vi "general query.vi"(0 "VISA resource name":refnum<visa-resource-name>="GPIB0::21::INSTR", 11 "error in (no error)":errorcluster) -> (2 "Range W and dBm":T3, 3 "In Range?":T2, 4 "VISA resource name out":refnum<visa-resource-name>, 6 "Power":string, 8 "Power num":dbl, 10 "Units":string, 13 "Averaging":T4, 14 "Auto Ranging?":T1, 15 "error out":errorcluster)   [LabVIEW 2017]
uses:
  Averaging control.ctl
  Range control watts and dBm.ctl
  Range Status.ctl
  Auto Range control.ctl
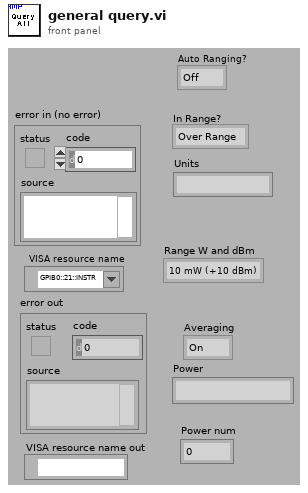
[diagram p1: front panel]
types:
  T1 = typedef "Auto Range control.ctl" = enum16{"Off", "On"}
  T2 = typedef "Range Status.ctl" = enum16{"Over Range", "Under Range", "In Range"}
  T3 = typedef "Range control watts and dBm.ctl" = enum16{"10 mW (+10 dBm)", "1 mW (0 dBm)", "100 uW (-10 dBm)", "10 uW (-20 dBm)", "1 uW (-30 dBm)", "100 nW (-40 dBm)", "10 nW (-50 dBm)", "1 nW (-60 dBm)", "100 pW (-70 dBm)", "10 pW (-80 dBm)"}
  T4 = typedef "Averaging control.ctl" = enum16{"On", "Off"}
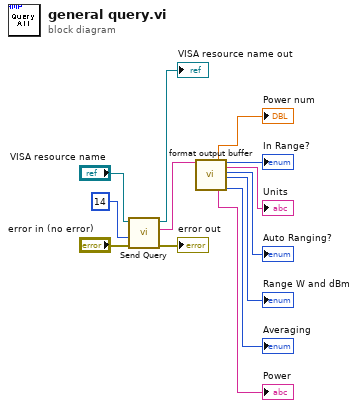
[diagram p0: block diagram]
diagram:
  n1 = call "Send Query.vi"("error in (no error)"="error in (no error)", "Bytes Count"=14, "VISA resource name"="VISA resource name") -> ("error out"=→"error out":errorcluster, "read buffer"=w8:string, "VISA resource name out"=→"VISA resource name out":refnum<visa-resource-name>)  [unwired: 6 in]
  n2 = call "format output buffer.vi"("read buffer"=w8) -> ("Power num"=→"Power num":dbl, "Power"=→"Power":string, "In Range?"=→"In Range?":T2, "Units"=→"Units":string, "Auto Ranging?"=→"Auto Ranging?":T1, "Range W/dBm"=→"Range W and dBm":T3, "Averaging"=→"Averaging":T4)  [unwired: 12 in]
